vi "IDByteToNotes.vi"(1 "ID Byte":i32=138) -> (0 "Notes":string)   [LabVIEW 2010]
doc: "Donne une explication du type de la donnée en fonction de son type de donnée"
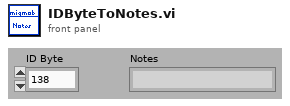
[diagram p1: front panel]
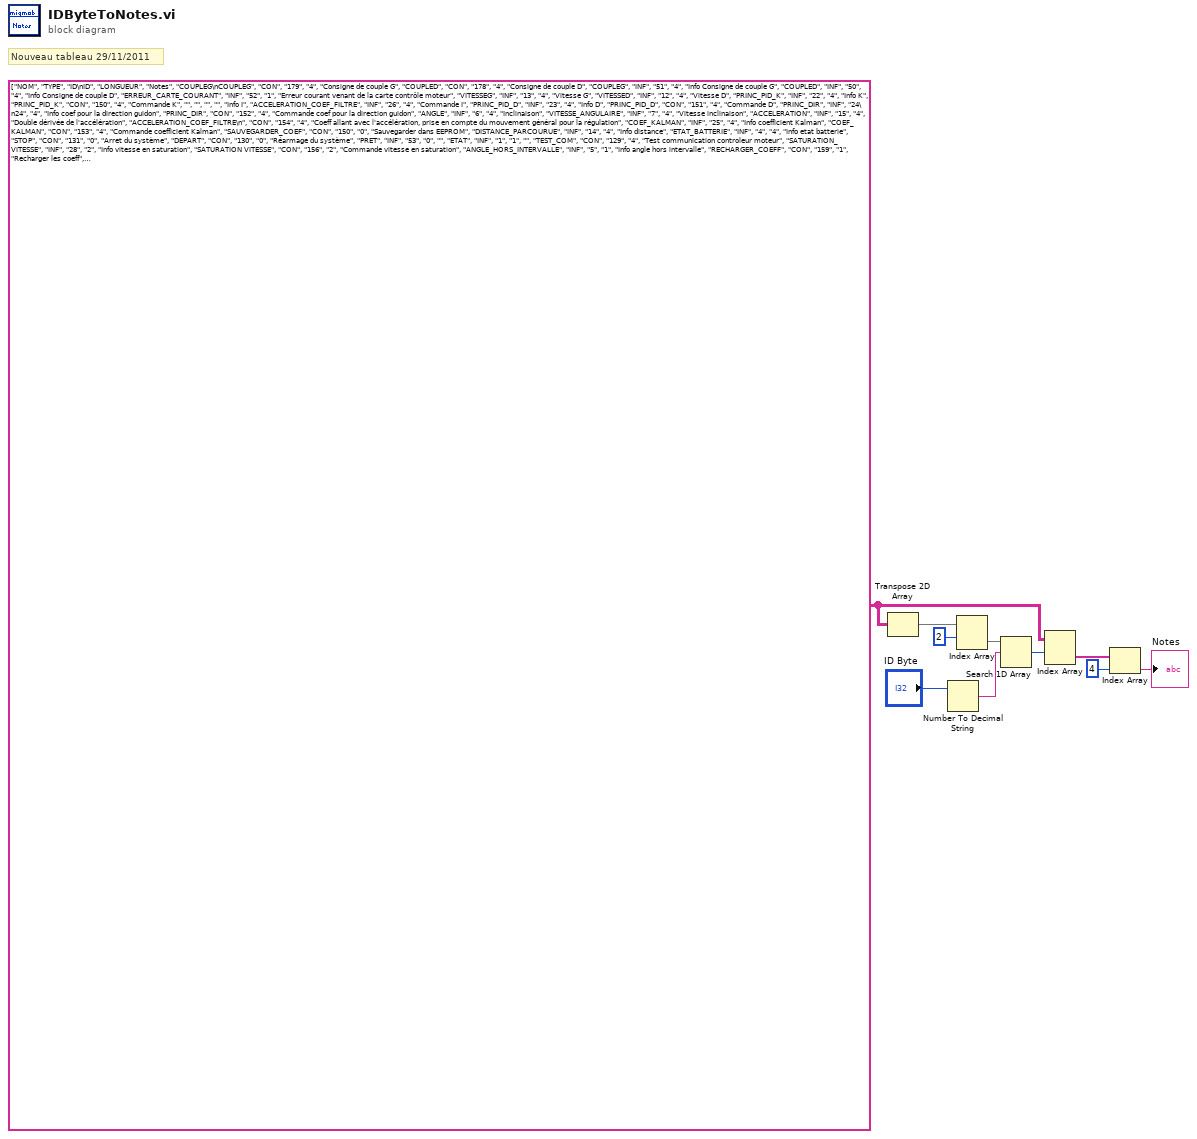
[diagram p0: block diagram]
diagram:
  w1 = string[][] [["NOM", "TYPE", "ID\nID", "LONGUEUR", "Notes"], ["COUPLEG\nCOUPLEG", "CON", "179", "4", "Consigne de couple G"], ["COUPLED", "CON", "178", "4", "Consigne de couple D"], ["COUPLEG", "INF", "51", "4", "Info Consigne de couple G"], ["COUPLED", "INF", "50", "4", "Info Consigne de couple D"], ["ERREUR_CARTE_COURANT", "INF", "52", "1", "Erreur courant venant de la carte contrôle moteur"], ["VITESSEG", "INF", "13", "4", "Vitesse G"], ["VITESSED", "INF", "12", "4", "Vitesse D"], ["PRINC_PID_K", "INF", "22", "4", "Info K"], ["PRINC_PID_K", "CON", "150", "4", "Commande K"], ["", "", "", "", "Info I"], ["ACCELERATION_COEF_FILTRE", "INF", "26", "4", "Commande I"], ["PRINC_PID_D", "INF", "23", "4", "Info D"], ["PRINC_PID_D", "CON", "151", "4", "Commande D"], ["PRINC_DIR", "INF", "24\n24", "4", "Info coef pour la direction guidon"], ["PRINC_DIR", "CON", "152", "4", "Commande coef pour la direction guidon"], ["ANGLE", "INF", "6", "4", "Inclinaison"], ["VITESSE_ANGULAIRE", "INF", "7", "4", "Vitesse inclinaison"], ["ACCELERATION", "INF", "15", "4", "Double dérivée de l'accélération"], ["ACCELERATION_COEF_FILTRE\n", "CON", "154", "4", "Coeff allant avec l'accélération, prise en compte du mouvement général pour la régulation"], ["COEF_KALMAN", "INF", "25", "4", "Info coefficient Kalman"], ["COEF_KALMAN", "CON", "153", "4", "Commande coefficient Kalman"], ["SAUVEGARDER_COEF", "CON", "150", "0", "Sauvegarder dans EEPROM"], ["DISTANCE_PARCOURUE", "INF", "14", "4", "Info distance"], ["ETAT_BATTERIE", "INF", "4", "4", "Info etat batterie"], ["STOP", "CON", "131", "0", "Arret du système"], ["DEPART", "CON", "130", "0", "Réarmage du système"], ["PRET", "INF", "53", "0", ""], ["ETAT", "INF", "1", "1", ""], ["TEST_COM", "CON", "129", "4", "Test communication controleur moteur"], ["SATURATION_VITESSE", "INF", "28", "2", "Info vitesse en saturation"], ["SATURATION VITESSE", "CON", "156", "2", "Commande vitesse en saturation"], ["ANGLE_HORS_INTERVALLE", "INF", "5", "1", "Info angle hors intervalle"], ["RECHARGER_COEFF", "CON", "159", "1", "Recharger les coeff"], ["VERBOSE", "INF", "8", "2", ""], ["VERBOSE", "CON", "136", "2", ""], ["DEMANDE_COEFFICIENTS", "CON", "137", "1", ""], ["CHARGER_VITESSE", "CON", "144", "0", ""], ["ENREGISTRER_VITESSE", "CON", "145", "0", ""], ["CHARGER_ASSERVISSEMENT", "CON", "146", "0", ""], ["ENREGISTRER_ASSERVISSEMENT", "CON", "147", "0", ""], ["CHARGER_DEMARRAGE", "CON", "148", "0", ""], ["ENREGISTRER_DEMARRAGE", "CON", "149", "0", ""], ["GUIDONMAX", "INF", "27", "4", ""], ["LIMITE_DISTANCE_UTILISATEUR", "INF", "28", "4", ""], ["DEMARRAGE_TOL_ANGLE", "INF", "29", "4", ""], ["DEMARRAGE_TOL_GUIDON", "INF", "30", "4", ""], ["DEMARRAGE_DELAI_EQUILIBRE", "INF", "31", "4", ""], ["VITESSE_TROTTOIR_MAX", "INF", "32", "4", ""], ["POURCENT_SECURITE_MOTEUR", "INF", "33", "4", ""], ["COEF_HYSTERESIS_SECURITE", "INF", "34", "4", ""], ["COEF_COURANT_1", "CON", "163", "4", ""], ["COEF_COURANT_1", "INF", "35", "4", ""], ["COEF_COURANT_2", "CON", "164", "4", ""], ["COEF_COURANT_2", "INF", "36", "4", ""]]
  # "Nouveau tableau 29/11/2011"
  n1 = Transpose 2D Array(2D array=w1) -> (transposed array=w2:string[][])
  n2 = Number To Decimal String(number="ID Byte") -> (decimal integer string=w6:string)  [unwired: 1 in]
  n3 = Index Array(array=w2, index (row)=2 ("indice (ligne)")) -> (element=w5:string[])  [unwired: 1 in]
  n4 = Search 1D Array(1D array=w5, element=w6) -> (index of element=w8:i32)  [unwired: 1 in]
  n5 = Index Array(array=w1, index (row)=w8) -> (element=w4:string[])  [unwired: 1 in]
  n6 = Index Array(array=w4, index=4 ("indice")) -> (element=→"Notes":string)
